vi "byte_expand_ads1293.vi"() -> ()   [LabVIEW 2013]
uses:
  <vilib>/Analysis/3filter.llb/Filter Passband Type.ctl
  <vilib>/Instr/_visa.llb/VISA Configure Serial Port (Instr).vi
  <vilib>/Analysis/3filter.llb/Butterworth Filter (DBL).vi
  <vilib>/measure/maspectr.llb/FFT Power Spectrum and PSD for 1 Chan.vi
  <vilib>/measure/maspectr.llb/FFT Power Spectrum for N Chan.vi
  <vilib>/measure/NI_MAPro.lvlib
  <vilib>/Analysis/NI_AALBase.lvlib
panel:
  in  "Полоса пропускания, Гц":dbl=250.0 format="%0.2f"
  out "Sleep Norm":bool
  out "PWR_OUT":T1(graph)
  in  "Порог":dbl(slide) scale=0.0..1500.0
  in  "averaging parameters":T2={"averaging mode"=enum."RMS averaging", "weighting mode"=enum."Exponential", "number of averages"=3} {"number of averages" min=1}
  in  "Канал":bool
  out "CH 2":waveform(dbl)(graph)
  in  "Запись":bool
  out "FFT":cluster{"f0":dbl, "df":dbl, "magnitude":dbl[]}(graph)
  in  "Заметка":string="Плата сбора данных основана на Atmega32\nАЦП ADS1293, частота дискретизации 2400 Гц.\nСимвольная скорость порта 230400 бод\nДополнительная информация:\n"
  in  "Рабочая папка для сохранения файлов":path=path "D:/АгеевВБ/СГУ/Научная_работа/ЭЭГ/Сон_звук/ээг_я"
  out "CH 1":waveform(dbl)(graph)
  in  "stop":bool
  in  "Порт":refnum<visa-resource-name>
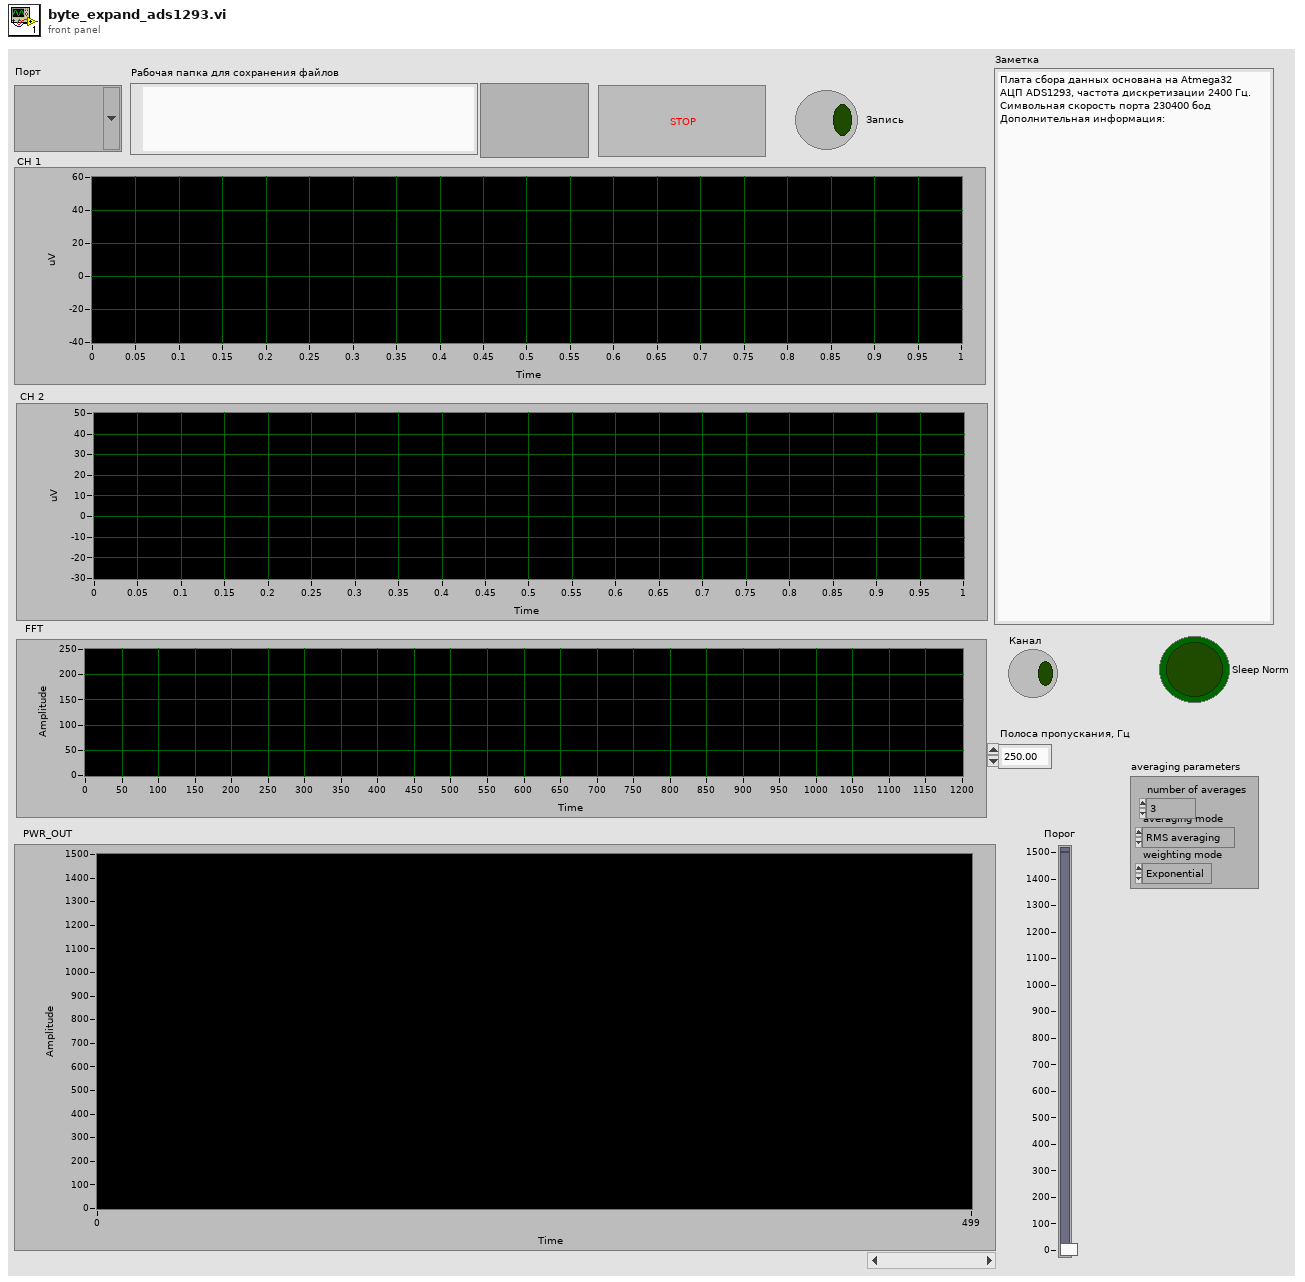
[diagram p1: front panel]
types:
  T1 = cluster{"PWR_BAND":dbl, "PWR_BAND":dbl, "PWR_BAND":dbl, "PWR_BAND":dbl, "Порог срабатывания":dbl, dbl, "Порог отсечки":dbl}
  T2 = cluster{"averaging mode":enum16{"No averaging", "Vector averaging", "RMS averaging", "Peak hold"}, "weighting mode":enum16{"Linear", "Exponential"}, "number of averages":u32}
  T3 = typedef "NI_AALBase.lvlib/Filter Passband Type.ctl" = enum32{"Lowpass", "Highpass", "Bandpass", "Bandstop"}
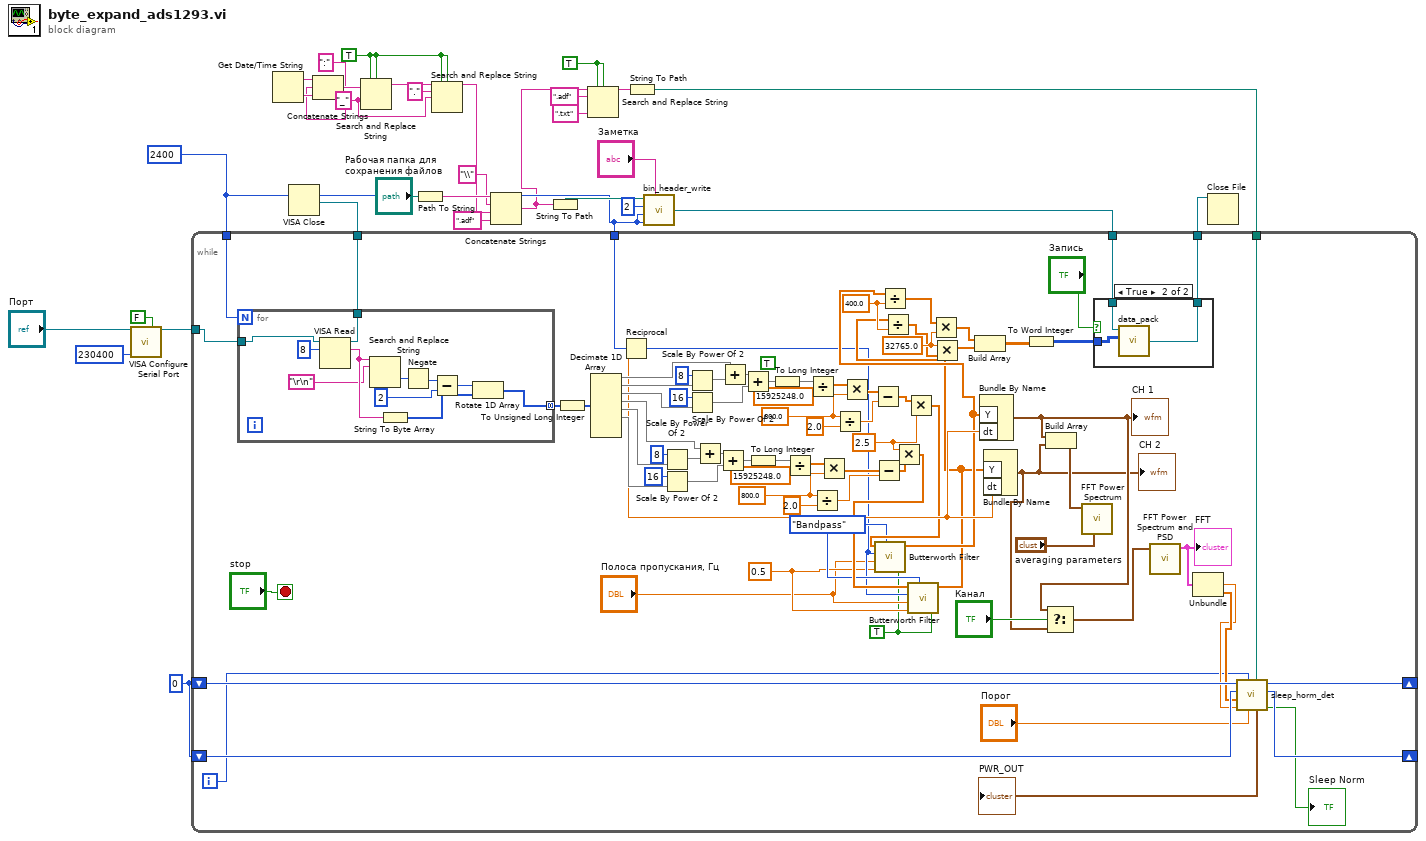
[diagram p0: block diagram]
diagram:
  w3 = TRUE ("replace all? (F)")
  w7 = 0 ("Shift_Out")
  w8 = i16 2400 ("-x")
  w13 = TRUE ("ignore case? (F)")
  w10 = "_" ("replace string (\"\")")
  n1 = call-poly "VISA Configure Serial Port"("VISA resource name"="Порт", "Enable Termination\nChar (T)"=FALSE ("Enable Termination\nChar (T)"), "baud rate (9600)"=u32 230400) -> ("VISA resource name out"=w9:refnum<visa-resource-name>)  [unwired: 11 in, 1 out]
  n2 = Get Date/Time String() -> (date string=w18:string, time string=w11:string)  [unwired: 3 in]
  n3 = Concatenate Strings(w18, w10, w11) -> (w17:string)
  n4 = Search and Replace String(replace all?=w13, case sensitive?=w13, input string=w17, search string=":", replace string=w10) -> (result string=w15:string)  [unwired: 3 in, 3 out]
  n5 = Path To String(path="Рабочая папка для сохранения файлов") -> (string=w26:string)
  n6 = Search and Replace String(replace all?=w13, case sensitive?=w13, input string=w15, search string=".", replace string=w10) -> (result string=w12:string)  [unwired: 3 in, 3 out]
  n7 = Concatenate Strings(w26, "\\" ("string"), w12, ".adf" ("string")) -> (w6:string)
  n8 = String To Path(string=w6) -> (path=w23:path)
  n9 = Search and Replace String(replace all?=w3, case sensitive?=w3, input string=w6, search string=".adf", replace string=".txt" ("replace string (\"\")")) -> (result string=w2:string)  [unwired: 3 in, 3 out]
  n10 = String To Path(string=w2) -> (path=w1:path)
  n11 = call "bin_header_write.vi"("New_BIN_FILE"=w23, "CH_NUM"=u8 2, "Length"=w8, "Freq_d"=w8, "Meta"="Заметка") -> ("refnum_out"=w21:refnum<file>)
  n12 = while {
    tunnel: [w111] -> w29
    tunnel: w21 -> [w94]
    tunnel: w8 -> [w38]
    tunnel: w8 -> [w95]
    tunnel: [w93] -> w19
    tunnel: w9 -> [w76]
    shift-right: [w56] -> _
    shift-left: w7 -> [w57]
    shift-right: [w55] -> _
    shift-left: w7 -> [w54]
    tunnel: w1 -> [w47]
    i -> [w48]
    stop <- "stop" stop-if-true
    w35 = TRUE ("init/cont (init:F)")
    w37 = 0.5 ("low cutoff freq: fl")
    w39 = Filter_Passband_Type."Bandpass" ("filter type")
    w45 = 2.5 ("y")
    w68 = 400.0 ("y")
    w69 = 32765.0 ("x")
    w81 = 800.0 ("y")
    w87 = 800.0 ("y")
    (unwired) TRUE ("init/cont (init:F)")
    n13 = for {
      N: w95 -> [_]
      tunnel: w76 -> [w116]
      tunnel: [w126] -> w111
      tunnel: [w117] -> w109 mode=concatenating
      n14 = VISA Read(VISA resource name=w116, byte count=u32 8) -> (VISA resource name out=w126:refnum<visa-resource-name>, read buffer=w123:string)  [unwired: 1 in, 2 out]
      n15 = Search and Replace String(input string=w123, search string="\r\n") -> (offset past replacement=w121:i32)  [unwired: 6 in, 3 out]
      n16 = String To Byte Array(string=w123) -> (unsigned byte array=w124:u8[])
      n17 = Negate(x=w121) -> (-x=w120:i32)
      n18 = Subtract(x=w120, y=2 ("-x")) -> (x-y=w118:i32)
      n19 = Rotate 1D Array(1:w124, 2:w118) -> (0:w117:u8[])
    }
    n20 = To Unsigned Long Integer(number=w109) -> (unsigned 32bit integer=w108:u32[])
    n21 = Decimate 1D Array(w108) -> (w101:u32[], w106:u32[], w104:u32[], w72:u32[], w71:u32[], w70:u32[])  [unwired: 2 out]
    n22 = Reciprocal(x=w38) -> (1/x=w65:dbl)
    n23 = Scale By Power Of 2(n=i16 8, x=w71) -> (x*2^n=w97:u32[])
    n24 = Scale By Power Of 2(n=i16 16, x=w70) -> (x*2^n=w73:u32[])
    n25 = Scale By Power Of 2(n=i16 8, x=w106) -> (x*2^n=w102:u32[])
    n26 = Scale By Power Of 2(n=i16 16, x=w104) -> (x*2^n=w74:u32[])
    n27 = Add(x=w72, y=w97) -> (x+y=w96:u32[])
    n28 = Add(x=w96, y=w73) -> (x+y=w78:u32[])
    n29 = Add(x=w101, y=w102) -> (x+y=w100:u32[])
    n30 = Add(x=w100, y=w74) -> (x+y=w92:u32[])
    n31 = To Long Integer(number=w78) -> (32bit integer=w77:i32[])
    n32 = To Long Integer(number=w92) -> (32bit integer=w90:i32[])
    n33 = Divide(x=w77, y=15925248.0) -> (x/y=w83:dbl[])
    n34 = Divide(x=w90, y=15925248.0) -> (x/y=w89:dbl[])
    n35 = Divide(x=w81, y=2.0) -> (x/y=w79:dbl)
    n36 = Multiply(x=w83, y=w81) -> (x*y=w82:dbl[])
    n37 = Divide(x=w87, y=2.0) -> (x/y=w85:dbl)
    n38 = Multiply(x=w89, y=w87) -> (x*y=w88:dbl[])
    n39 = Subtract(x=w88, y=w85) -> (x-y=w46:dbl[])
    n40 = Subtract(x=w82, y=w79) -> (x-y=w44:dbl[])
    n41 = Multiply(x=w45, y=w44) -> (x*y=w41:dbl[])
    n42 = Multiply(x=w46, y=w45) -> (x*y=w43:dbl[])
    n43 = call-poly <vilib>:"Butterworth Filter.vi"("init/cont (init:F)"=w35, "filter type"=w39, "low cutoff freq: fl"=w37, "high cutoff freq: fh"="Полоса пропускания, Гц", "sampling freq: fs"=w38, "X"=w43) -> ("Filtered X"=w42:dbl[])  [unwired: 2 in, 1 out]
    n44 = Divide(x=w42, y=w68) -> (x/y=w66:dbl[])
    n45 = call-poly <vilib>:"Butterworth Filter.vi"("init/cont (init:F)"=w35, "filter type"=w39, "low cutoff freq: fl"=w37, "high cutoff freq: fh"="Полоса пропускания, Гц", "sampling freq: fs"=w38, "X"=w41) -> ("Filtered X"=w40:dbl[])  [unwired: 2 in, 1 out]
    n46 = Divide(x=w40, y=w68) -> (x/y=w67:dbl[])
    n47 = Multiply(x=w66, y=w69) -> (x*y=w34:dbl[])
    n48 = Multiply(x=w69, y=w67) -> (x*y=w33:dbl[])
    n49 = Build Array(w34, w33) -> (w32:dbl[][])
    n50 = Bundle By Name("Y"=w42, "dt"=w65) -> (w60:waveform(dbl))  [unwired: 1 in]
    "CH 1" <- w60
    n51 = Bundle By Name("Y"=w40, "dt"=w65) -> (w59:waveform(dbl))  [unwired: 1 in]
    "CH 2" <- w59
    n52 = To Word Integer(number=w32) -> (16bit integer=w75:i16[][])
    n53 = Select(t=w60, s="Канал", f=w59) -> (s? t:f=w58:waveform(dbl))
    n54 = Build Array(w60, w59) -> (w63:waveform(dbl)[])
    n55 = call-poly <vilib>:"FFT Power Spectrum.vi"("averaging parameters"="averaging parameters", "time signals"=w63) -> ()  [unwired: 6 in, 4 out]
    n56 = case shown="True" "Запись" {
      tunnel: w94 -> [w112 w115]
      tunnel: [w112 w114] -> w93
      tunnel: w75 -> [_ w113]
      frame False {
      }
      frame True {
        n57 = call "data_pack.vi"("in_data"=w113, "refnum_in"=w115) -> ("refnum_out"=w114:refnum<file>)  [unwired: 2 in]
      }
    }
    n58 = call-poly <vilib>:"FFT Power Spectrum and PSD.vi"("time signal"=w58) -> ("Power Spectrum / PSD"=w64:cluster{"f0":dbl, "df":dbl, "magnitude":dbl[]})  [unwired: 7 in, 3 out]
    "FFT" <- w64
    n59 = Unbundle(w64) -> ("df"=w52:dbl, "magnitude"=w53:dbl[])  [unwired: 1 out]
    n60 = call "sleep_horm_det.vi"("Path_Sleep_list"=w47, "Порог срабатывания"="Порог", "sec_in"=w48, "df"=w52, "Спектр ЭЭГ сигнала"=w53, "Shift_Amp_in"=w54, "Shift_Sleep_in"=w57) -> ("Sleep Norm"=→"Sleep Norm":bool, "Shift_Amp_out"=w55:u16, "Shift_Sleep_out"=w56:i32, "Индексы мощности"=→"PWR_OUT":T1)  [unwired: 1 in]
  }
  n61 = VISA Close(VISA resource name=w29) -> ()  [unwired: 1 in, 1 out]
  n62 = Close File(refnum=w19) -> ()  [unwired: 1 in, 2 out]
